vi "Metadata From Server.vi"(8 "error in (no error)":errorcluster, 11 "Log Record in":refnum<class "Log Record.lvclass">) -> (0 "error out":errorcluster, 3 "Log Record out":refnum<class "Log Record.lvclass">)   [LabVIEW 2020, in "Log Record.lvclass"]
uses:
  Log Record.lvclass
  NHMFL_Core/Libraries/FAIR Data/MagX/Experiment info.ctl
  Log Record.lvclass/Log Record.ctl
panel:
  out "Data out":T1[](array[typedef])
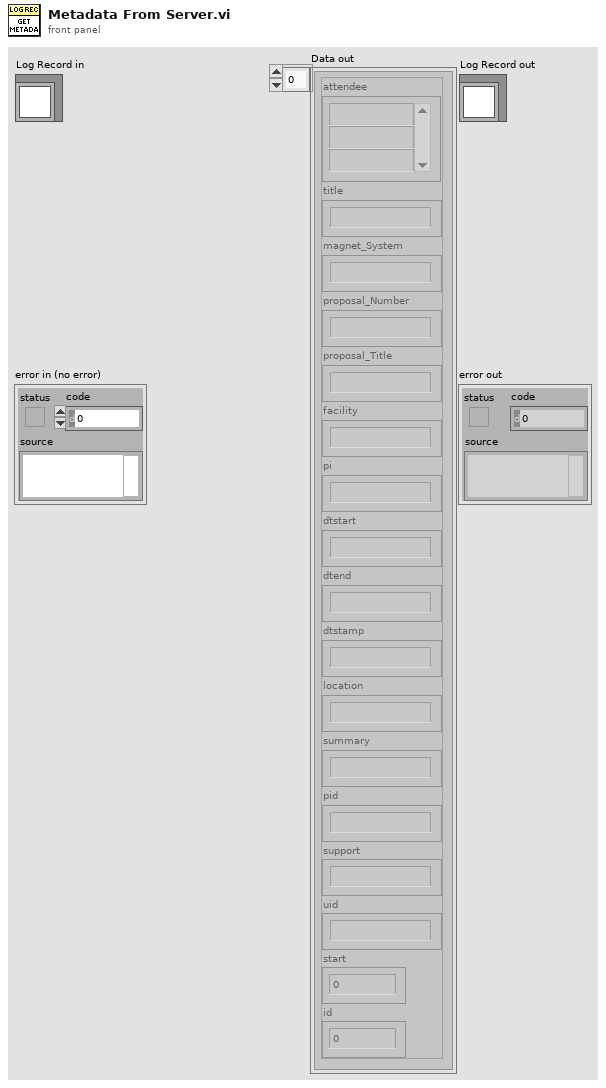
[diagram p1: front panel]
types:
  T1 = typedef "Experiment info.ctl" = cluster{"attendee":string[], "title":string, "magnet_System":string, "proposal_Number":string, "proposal_Title":string, "facility":string, "pi":string, "dtstart":string, "dtend":string, "dtstamp":string, "location":string, "summary":string, "pid":string, "support":string, "uid":string, "start":u64, "id":u64}
  T2 = typedef "Log Record Configuration.ctl" = cluster{"OSF node  ID":string, "Conection timeout":dbl, "Station":string, "Log server ":string, "Upload to OSF":bool, "Append to lab book":bool, "Filing moduled":string[]}
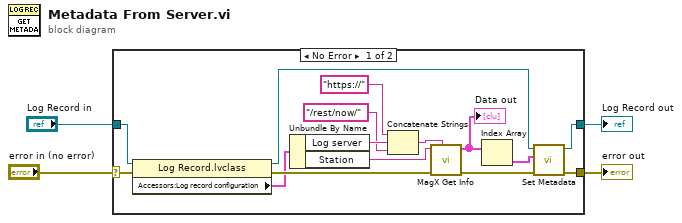
[diagram p0: block diagram]
diagram:
  n1 = case shown="No Error" "error in (no error)" {
    selector: "error in (no error)" -> [w19 w21]
    tunnel: [w5 w21] -> w3
    tunnel: [w9 w20] -> w1
    tunnel: "Log Record in" -> [w16 w20]
    frame No Error {
      n2 = property class="Log Record.lvclass"(reference=w16, error in=w19) -> (reference out=w7:refnum<class "Log Record.lvclass">, error out=w17:errorcluster, "Accessors:Log record configuration"=w15:T2)
      n3 = Unbundle By Name(w15) -> ("Log server"=w12:string, "Station"=w14:string)
      n4 = Concatenate Strings("https://" ("string"), w12, "/rest/now/" ("string")) -> (w10:string)
      n5 = call "MagX Get Info.vi"("url"=w10, "error in"=w17, "Station"=w14) -> ("error out"=w6:errorcluster, "Data out"=w18:T1[])  [unwired: 7 in]
      "Data out" <- w18
      n6 = Index Array(array=w18) -> (element=w8:T1)  [unwired: 1 in]
      n7 = call-dynamic "Set Metadata.vi"("error in (no error)"=w6, "Experiment info"=w8, "Log Record in"=w7) -> ("error out"=w5:errorcluster, "Log Record out"=w9:refnum<class "Log Record.lvclass">)  [unwired: 7 in]
    }
    frame Error {
    }
  }
  "error out" <- w3
  "Log Record out" <- w1
